vi "Module Init.vi"(8 "error in (no error)":errorcluster, 11 "Event Reporter Module in":refnum<class "Event Reporter Module.lvclass">) -> (0 "error out":errorcluster, 3 "Event Reporter Module out":refnum<class "Event Reporter Module.lvclass">)   [LabVIEW 2020, in "Volatus.lvlib" / "Event Reporter Module.lvclass"]
uses:
  Event Reporter Module.lvclass
  C:/dev/lv20CE/relink/lv-volatus/Volatus/Module/Module.lvclass
  Module/Module.lvclass/Module.ctl
  MessageQ/MessageQ.lvclass/MessageQ.ctl
  Module/Self Q.vi
  MessageQ/Send.vi
  Event Reporter Module.lvclass/Event Reporter Module.ctl
  Module/Module.lvclass
  C:/dev/lv20CE/relink/lv-volatus/Volatus/Event Reporter Module/Event Reporter Module.lvclass
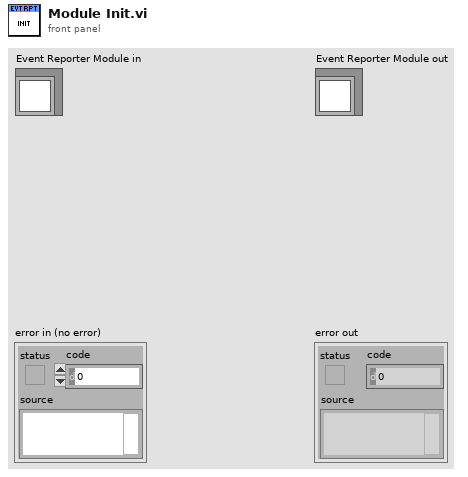
[diagram p1: front panel]
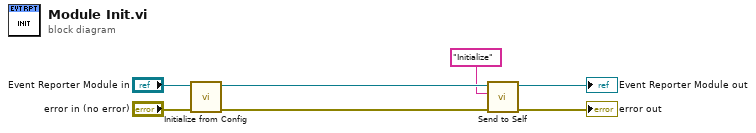
[diagram p0: block diagram]
diagram:
  n1 = call "Initialize from Config.vi"("error in (no error)"="error in (no error)", "Event Reporter Module in"="Event Reporter Module in") -> ("error out"=w3:errorcluster, "Event Reporter Module out"=w2:refnum<class "Event Reporter Module.lvclass">)  [unwired: 8 in]
  n2 = call "Send to Self.vi"("error in (no error)"=w3, "Message ID"="Initialize", "Module in"=w2) -> ("error out"=→"error out":errorcluster, "Module out"=→"Event Reporter Module out":refnum<class "Event Reporter Module.lvclass">)  [unwired: 7 in]
